vi "Write Background Image.vi"(5 "image data":T1, 9 "Pane in":refnum<class "Pane.lvclass">) -> (3 "Pane out":refnum<class "Pane.lvclass">)   [LabVIEW 2014, in "Pane.lvclass"]
uses:
  Pane.lvclass
  <vilib>/picture/picture.llb/imagedata.ctl
  Pane.lvclass/Pane.ctl
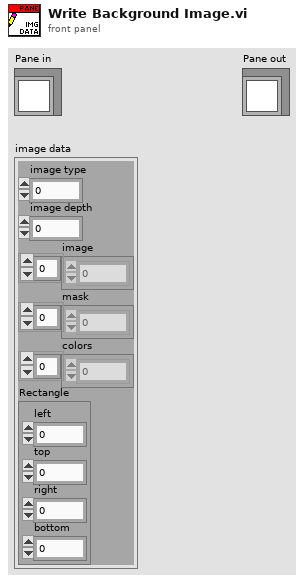
[diagram p1: front panel]
types:
  T1 = typedef "imagedata.ctl" = cluster{"image type":i32, "image depth":i32, "image":u8[], "mask":u8[], "colors":u32[], "Rectangle":cluster{"left":i16, "top":i16, "right":i16, "bottom":i16}}
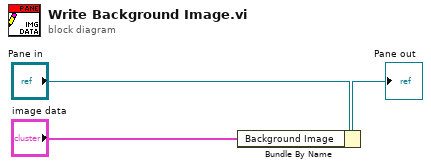
[diagram p0: block diagram]
diagram:
  n1 = Bundle By Name(cluster="Pane in", "Background Image"="image data") -> (→"Pane out":refnum<class "Pane.lvclass">)
